vi "Aumento Credito.vi"(8 "error in (no error)":errorcluster, 10 "Dinero":i32, 11 "Dinero in":refnum<class "Dinero.lvclass">) -> (0 "error out":errorcluster, 3 "Dinero out":refnum<class "Dinero.lvclass">)   [LabVIEW 2020, in "Dinero.lvlib" / "Dinero.lvclass"]
uses:
  Dinero.lvclass
  C:/Program Files (x86)/National Instruments/LabVIEW 2020/vi.lib/ActorFramework/Actor/Actor.lvclass
  Dinero.lvclass/Dinero.ctl
  <vilib>/ActorFramework/Actor/Actor.lvclass/Actor.ctl
  UI Messages/Obtain Credito from Dinero Msg/Obtain Credito from Dinero Msg.lvclass/Obtain Credito from Dinero Msg.ctl
  <vilib>/ActorFramework/Message Enqueuer/Message Enqueuer.lvclass/Message Enqueuer.ctl
  <vilib>/ActorFramework/Message Enqueuer/Enqueue.vi
  UI Messages/Obtain Credito from Dinero Msg/Obtain Credito from Dinero Msg.lvclass
  C:/Program Files (x86)/National Instruments/LabVIEW 2020/vi.lib/ActorFramework/Message/Message.lvclass
  <vilib>/ActorFramework/Message Priority Queue/Priority Enqueue.vi
  <vilib>/ActorFramework/Actor/Actor.lvclass
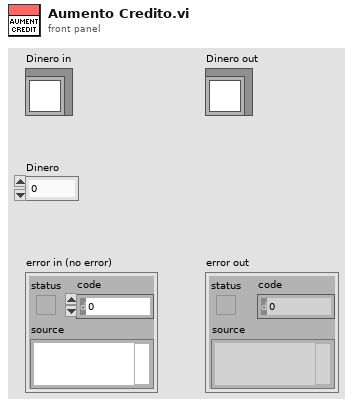
[diagram p1: front panel]
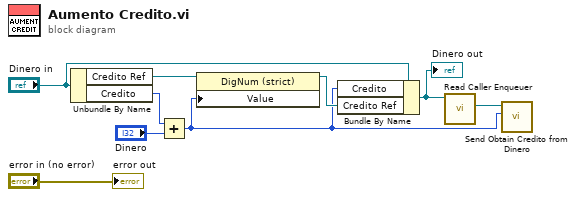
[diagram p0: block diagram]
diagram:
  n1 = Unbundle By Name("Dinero in") -> ("Credito Ref"=w8:refnum<vi>, "Credito"=w6:i32)
  n2 = Add(x=w6, y="Dinero") -> (x+y=w1:i32)
  n3 = property class="DigNum (strict)"(reference=w8, "Value"=w1) -> (reference out=w7:refnum<vi>)  [unwired: 1 in, 1 out]
  n4 = Bundle By Name(cluster="Dinero in", "Credito"=w1, "Credito Ref"=w7) -> (w3:refnum<class "Dinero.lvclass">)
  "Dinero out" <- w3
  n5 = call <vilib>:"Read Caller Enqueuer.vi"("Actor"=w3) -> ("Caller Enqueuer"=w2:refnum<class "Message Enqueuer.lvclass">)  [unwired: 10 in]
  n6 = call "Send Obtain Credito from Dinero.vi"("Credito"=w1, "Message Enqueuer"=w2) -> ()  [unwired: 8 in, 2 out]
  "error out" <- "error in (no error)"
